vi "Instrument Do Core.vi"(8 "error in (no error)":errorcluster, 9 "Instrument in":refnum<class "Instrument Driver.lvclass">, 10 "Actor in":refnum<class "Actor.lvclass">, 11 "Test Instrument Msg in":refnum<class "Test Instrument Msg.lvclass">) -> (0 "error out":errorcluster, 1 "Instrument out":refnum<class "Instrument Driver.lvclass">, 2 "Actor out":refnum<class "Actor.lvclass">, 3 "Test Instrument Msg out":refnum<class "Test Instrument Msg.lvclass">, 5 "Data":refnum<class "Data.lvclass">)   [LabVIEW 2020, in "Test.lvlib" / "Test Instrument Msg.lvclass"]
uses:
  Test Instrument Msg.lvclass
  PPL/HDH.Actor Framework.Core.Actor.lvlibp/1abvi3w/vi.lib/ActorFramework/Actor/Actor.lvclass
  PPL/HDH.Data.Generic.lvlibp/Data.lvclass
  PPL/HDH.Actor Framework.Core.Instrument Driver.lvlibp/Instrument Driver/Instrument Driver.lvclass
  Instrument/Test Instrument/Test Instrument.lvclass
  C:/Current projects/WS/PPL/HDH.Actor Framework.Core.Instrument Driver.lvlibp/Instrument Driver/Instrument Driver.lvclass
  Data/Test Double Data/Test Double Data.lvclass/Test Double Data.ctl
  Data/Test Double Data/Test Double Data.lvclass
  C:/Current projects/WS/PPL/HDH.Data.Generic.lvlibp/Data.lvclass
  PPL/HDH.Actor Framework.Core.Instrument Handler.lvlibp/Messages/Instrument Msg/Instrument Msg.lvclass
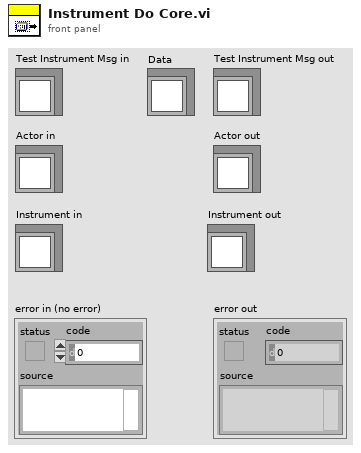
[diagram p1: front panel]
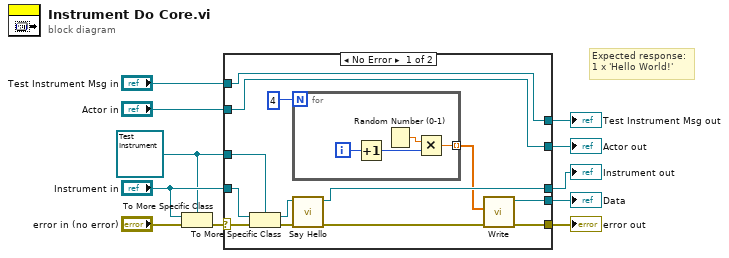
[diagram p0: block diagram]
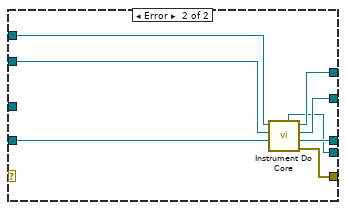
[diagram p2: hidden frame]
diagram:
  w1 = refnum<class "Test Instrument.lvclass"> refnum ("Test.lvlib:Test Instrument.lvclass")
  # "Expected response:\n1 x 'Hello World!'"
  n1 = To More Specific Class(target class=w1, reference="Instrument in", error in="error in (no error)") -> (error out=w3:errorcluster)  [unwired: 1 out]
  n2 = case shown="No Error" w3 {
    selector: w3 -> [w24 _]
    tunnel: [w15 w36] -> w11
    tunnel: [w19 w35] -> w10
    tunnel: [w18 w34] -> w9
    tunnel: [w17 w33] -> w8
    tunnel: [w14 w32] -> w7
    tunnel: "Actor in" -> [w18 w31]
    tunnel: "Test Instrument Msg in" -> [w17 w30]
    tunnel: "Instrument in" -> [w23 w29]
    tunnel: w1 -> [w22 _]
    frame No Error {
      n3 = To More Specific Class(target class=w22, reference=w23, error in=w24) -> (specific class reference=w21:refnum<class "Test Instrument.lvclass">, error out=w20:errorcluster)
      n4 = for {
        N: 4 -> [_]
        tunnel: [w25] -> w12 mode=indexing
        i -> [w27]
        n5 = Increment(x=w27) -> (x+1=w26:i32)
        n6 = Random Number (0-1)() -> (number: 0 to 1=w28:dbl)
        n7 = Multiply(x=w28, y=w26) -> (x*y=w25:dbl)
      }
      n8 = call "Say Hello.vi"("error in (no error)"=w20, "Test Instrument in"=w21) -> ("error out"=w16:errorcluster, "Test Instrument out"=w19:refnum<class "Test Instrument.lvclass">)  [unwired: 8 in]
      n9 = call "Write.vi"("error in (no error)"=w16, "Data"=w12) -> ("error out"=w15:errorcluster, "Test Double Data out"=w14:refnum<class "Test Double Data.lvclass">)  [unwired: 8 in]
    }
    frame Error {
      n10 = call-parent "Instrument Do Core.vi"("Instrument in"=w29, "Actor in"=w31, "Instrument Msg in"=w30) -> ("error out"=w36:errorcluster, "Instrument out"=w35:refnum<class "Instrument Driver.lvclass">, "Actor out"=w34:refnum<class "Actor.lvclass">, "Instrument Msg out"=w33:refnum<class "Test Instrument Msg.lvclass">, "Data"=w32:refnum<class "Data.lvclass">)  [unwired: 4 in]
    }
  }
  "error out" <- w11
  "Test Instrument Msg out" <- w8
  "Actor out" <- w9
  "Data" <- w7
  "Instrument out" <- w10
